vi "Read pointer.vi"(8 "error in (no error)":errorcluster, 11 "POSIX Thread Object in":refnum<class "POSIX Thread Object.lvclass">) -> (0 "error out":errorcluster, 2 "pointer":u64, 3 "POSIX Thread Object out":refnum<class "POSIX Thread Object.lvclass">)   [LabVIEW 2013, in "Linux RT IPC.lvlib" / "POSIX Threads.lvlib" / "POSIX Thread Object.lvclass"]
uses:
  POSIX Thread Object.lvclass
  POSIX Thread Object.lvclass/POSIX Thread Object.ctl
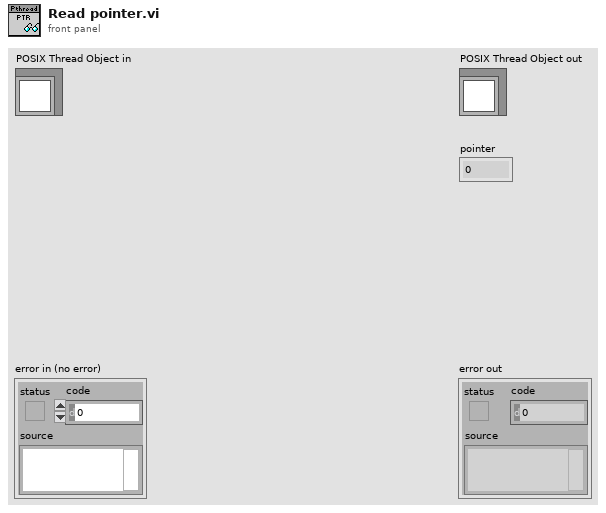
[diagram p1: front panel]
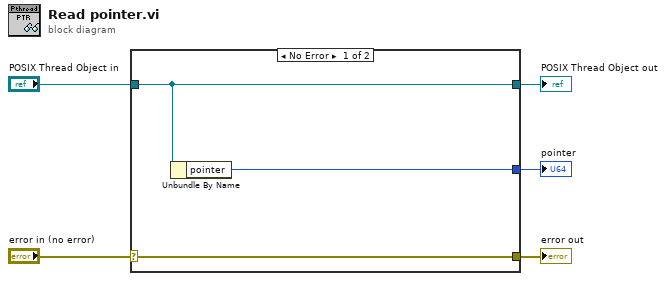
[diagram p0: block diagram]
diagram:
  n1 = case shown="No Error" "error in (no error)" {
    selector: "error in (no error)" -> [w8 w9]
    tunnel: [w8 w9] -> w4
    tunnel: [w7 w10] -> w2
    tunnel: "POSIX Thread Object in" -> [w7 w10]
    tunnel: [w6 _] -> w1
    frame No Error {
      n2 = Unbundle By Name(w7) -> ("pointer"=w6:u64)
    }
    frame Error {
    }
  }
  "error out" <- w4
  "POSIX Thread Object out" <- w2
  "pointer" <- w1
